vi "ROS Connection.vi"() -> ()   [LabVIEW 2020]
uses:
  <userlib>/ROS for LabVIEW Software/ROS/Code/Console/Servers/ServerSubs/TopicDef.ctl
  <userlib>/ROS for LabVIEW Software/ROS/Code/SubVIs/_ROSDirection.ctl
panel:
  out "error out":errorcluster
  in  "stop":bool
  out "Point":cluster{"x":dbl, "y":dbl, "z":dbl}
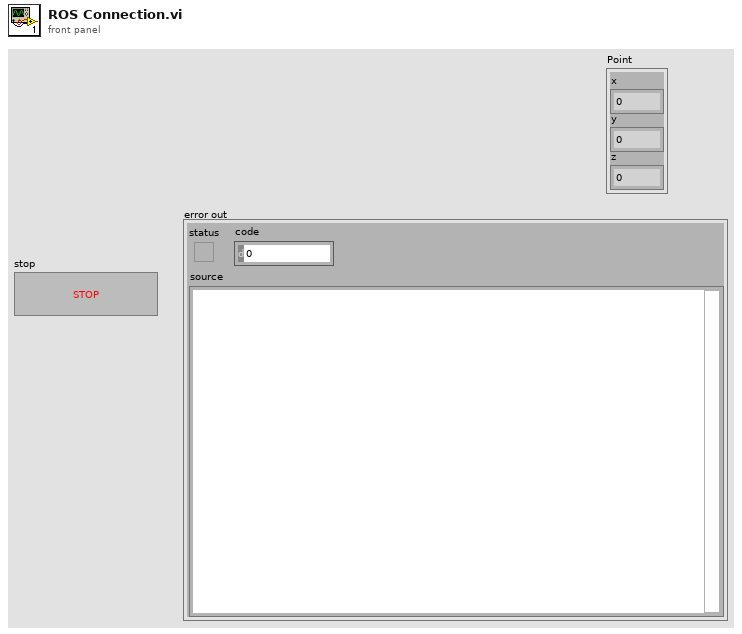
[diagram p1: front panel]
types:
  T1 = typedef "TopicDef.ctl" = cluster{"Topic":string, "Type":string, "Action":T2, "Update (ms)":u16, "queue size":u16}
  T2 = typedef "_ROSDirection.ctl" = enum16{"Node", "Publisher", "Subscriber", "ServiceClient", "ServiceProvider"}
  T3 = typedef "_ROSControl.ctl" = cluster{"topic port":u16, "Node":string, "topic":string, "type":string, "node port":u16, "error ":errorcluster, "Direction":T2, "Update (ms)":u16, "FIFO size":u16}
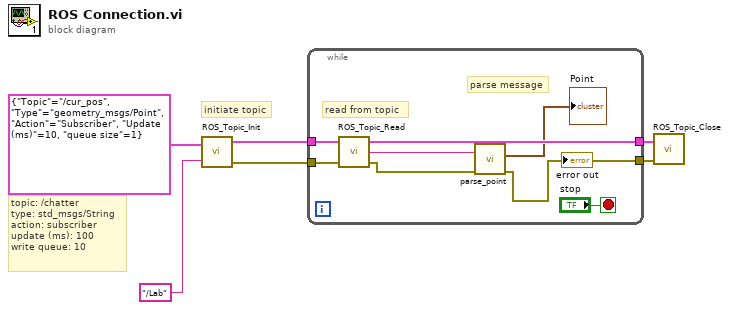
[diagram p0: block diagram]
diagram:
  # "initiate topic"
  # "topic: /chatter\ntype: std_msgs/String\naction: subscriber\nupdate (ms): 100\nwrite queue: 10"
  n1 = call <userlib>:"ROS_Topic_Init.vi"("Definitions"=T1 {"Topic"="/cur_pos", "Type"="geometry_msgs/Point", "Action"=enum."Subscriber", "Update (ms)"=10, "queue size"=1}, "node"="/Lab") -> ("ROS out"=w5:T3, "error out"=w4:errorcluster)  [unwired: 1 in]
  n2 = while {
    tunnel: w5 -> [w14]
    tunnel: w4 -> [w13]
    tunnel: [w11] -> w3
    tunnel: [w8] -> w2
    stop <- "stop" stop-if-true
    # "parse message"
    # "read from topic"
    n3 = call <userlib>:"ROS_Topic_Read.vi"("error in (no error)"=w13, "ROS in"=w14) -> ("error out"=w9:errorcluster, "Reply"=w10:string, "ROS out"=w11:T3)  [unwired: 1 in]
    n4 = call <userlib>:"parse_point.vi"("error in"=w9, "msg in"=w10) -> ("error out"=w8:errorcluster, "Point"=→"Point":cluster{"x":dbl, "y":dbl, "z":dbl})  [unwired: 3 in, 1 out]
    "error out" <- w8
  }
  n5 = call <userlib>:"ROS_Topic_Close.vi"("error in"=w2, "ROS in"=w3) -> ()  [unwired: 2 in, 1 out]
